vi "ScanParameters.vi"(9 "MainConfigurationArray":cluster{"Parameter":string, "Value":string}[](array[cluster]), 11 "Parameter":string) -> (3 "Value":string)   [LabVIEW 2017]
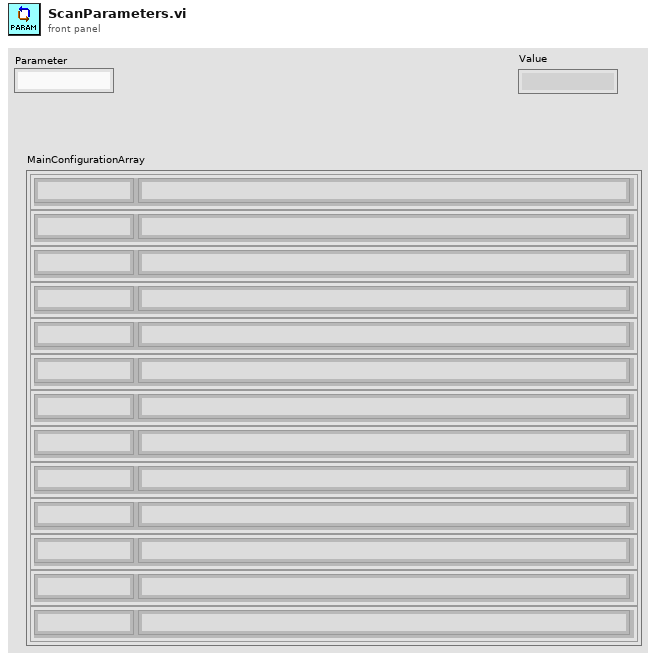
[diagram p1: front panel]
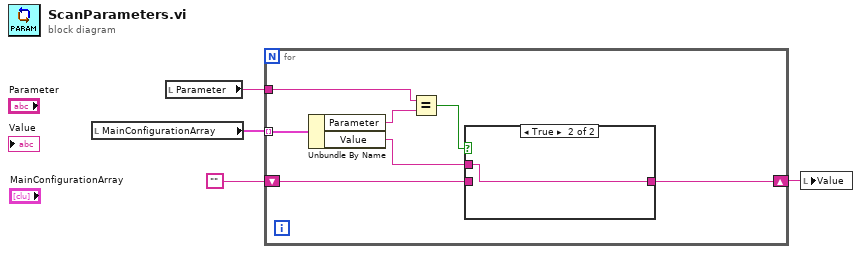
[diagram p0: block diagram]
diagram:
  n1 = local read "MainConfigurationArray"() -> (w1:cluster{"Parameter":string, "Value":string}[])
  n2 = local read "Parameter"() -> (w3:string)
  n3 = for {
    tunnel: w1 -> [w11] mode=indexing
    shift-right: [w6] -> w2
    shift-left: "" -> [w7]
    tunnel: w3 -> [w9]
    n4 = Unbundle By Name(w11) -> ("Parameter"=w10:string, "Value"=w5:string)
    n5 = Equal?(x=w9, y=w10) -> (x = y?=w8:bool)
    n6 = case shown="True" w8 {
      tunnel: [w12 w13] -> w6
      tunnel: w7 -> [w12 _]
      tunnel: w5 -> [_ w13]
      frame False {
      }
      frame True {
      }
    }
  }
  n7 = local write "Value"(w2) -> ()
